vi "BuildSavePath.vi"(10 "Meta Data":T1, 11 "Base path":path) -> (1 "ASCII Path":path, 2 "date/time string":string, 3 "XML Path":path)   [LabVIEW 2019]
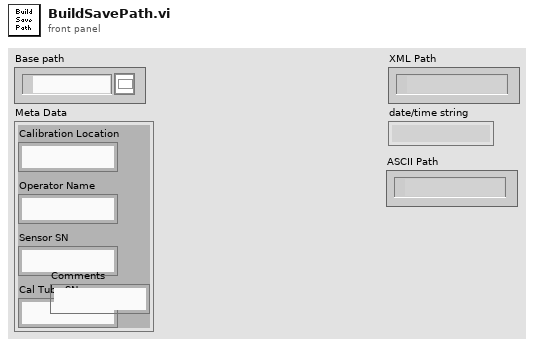
[diagram p1: front panel]
types:
  T1 = cluster{"Calibration Location":string, "Operator Name":string, "Sensor SN":string, "Cal Tube SN":string, "Comments":string}
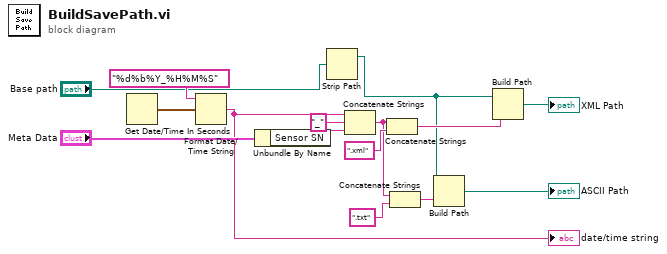
[diagram p0: block diagram]
diagram:
  n1 = Get Date/Time In Seconds() -> (seconds since 1Jan1904=w14:timestamp)
  n2 = Format Date/Time String(time format string (%c)="%d%b%Y_%H%M%S", seconds (now)=w14) -> (date/time string=w10:string)  [unwired: 1 in]
  "date/time string" <- w10
  n3 = Unbundle By Name("Meta Data") -> ("Sensor SN"=w12:string)
  n4 = Strip Path(path="Base path") -> (stripped path=w2:path)  [unwired: 1 out]
  n5 = Concatenate Strings(w10, "_" ("string"), w12) -> (w5:string)
  n6 = Concatenate Strings(w5, ".xml" ("string")) -> (w6:string)
  n7 = Concatenate Strings(w5, ".txt" ("string")) -> (w3:string)
  n8 = Build Path(base path=w2, name or relative path=w3) -> (appended path=→"ASCII Path":path)
  n9 = Build Path(base path=w2, name or relative path=w6) -> (appended path=→"XML Path":path)
